vi "McPherson Comm Globals.vi"() -> ()   [LabVIEW 2020]
uses:
  Serial Instruments/Serial Support VISA.llb/Communication Port.ctl
panel:
  in  "Max Slew [A/S]":dbl format="%.1f"
  in  "Max Current [kA]":dbl format="%.2f"
  in  "B=F(I)":dbl[](array[numeric])=[0.0, 1.0, 0.0] format="%.5e"
  in  "I=F(B)":dbl[](array[numeric])=[0.0, 1.0, 0.0] format="%.5e"
  in  "McP Communication Port":T1=1 items=["Modem", "Printer", "COM3", "COM4", "COM5", "COM6", "COM7", "COM8", "COM9", "Nothing", "LPT1", "LPT2", "LPT3", "LPT4"]
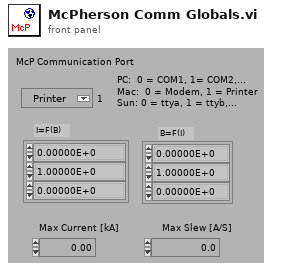
[diagram p1: front panel]
types:
  T1 = typedef "Communication Port.ctl" = u16
diagram:
